vi "send Command Response.vi"(0 "Listener Handle in":T1, 5 "REx Command":refnum<class "REx Command - Root.lvclass">, 11 "error in (no error)":errorcluster) -> (4 "Listener Handle out":T1, 15 "error out":errorcluster)   [LabVIEW 2012, in "REx.lvlib" / "Local Listener Session.lvclass"]
uses:
  Local Listener Session.lvclass
  Typedefs/Session Handle.ctl
  REx Command Root/REx Command - Root.lvclass
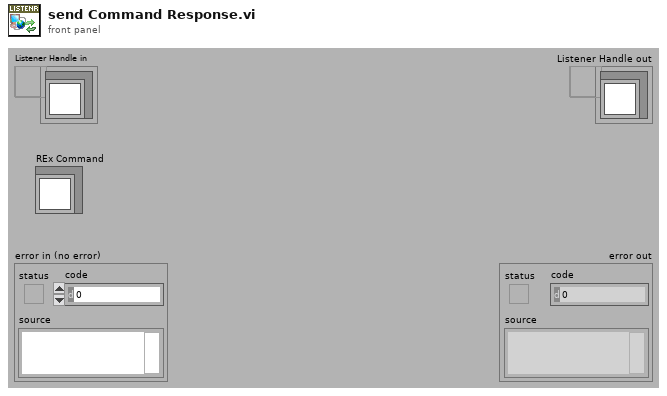
[diagram p1: front panel]
types:
  T1 = typedef "REx.lvlib/Local Listener Session.lvclass/Session Handle.ctl" = refnum<data-value>
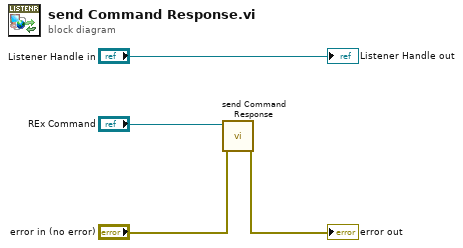
[diagram p0: block diagram]
diagram:
  n1 = call "send Command Response.vi"("error in (no error)"="error in (no error)", "REx Command - Root in"="REx Command") -> ("error out"=→"error out":errorcluster)  [unwired: 8 in, 1 out]
  "Listener Handle out" <- "Listener Handle in"
